vi "Memory.Pointer.External.Encapsulate.vi"(8 "error in (no error)":errorcluster, 10 "size":u64 format="%d bytes", 11 "address":u64 format="%016x") -> (0 "error out":errorcluster, 3 "external pointer":refnum<class "Memory.Pointer.External.lvclass">)   [LabVIEW 2016, in "Memory Manager.lvlib" / "Memory.Pointer.External.lvclass"]
doc: "Encapsulates an existing pointer allocated externally to LabVIEW to allow manipulation of that pointer using this library."
uses:
  Memory.Pointer.External.lvclass
  C:/Users/Ryan/Documents/Git/Sourcetree/LabVIEW-Memory-Manager/Source/Library/Classes/Pointer/Memory.Pointer.lvclass
  Pointer/Memory.Pointer.lvclass/Memory.Pointer.ctl
  Pointer/Methods/Memory.Pointer.Errors.vi
  Pointer/Methods/Memory.Pointer.Errors.Null Pointer.vi
  Pointer/Accessors/Get Address.vi
  Pointer/Methods/Memory.Pointer.Errors.Create Error.vi
  Submodules/Static Error Handling/Source/Library/VIs/Static Error Handling.Error Cluster Constant.vi
  Submodules/Static Error Handling/Source/Library/VIs/Static Error Handling.Error Cluster Constant (256B).vi
  Submodules/Static Error Handling/Source/Library/VIs/Static Error Handling.Parameters.Status.Set.vi
  Submodules/Static Error Handling/Source/Library/VIs/Static Error Handling.Parameters.Code.Set.vi
  Submodules/Static Error Handling/Source/Library/VIs/Static Error Handling.Parameters.VI Source.Set.vi
  Constants/Memory.Constants.vi
  Constants/Memory.Constants.Library Name.vi
  Pointer/Methods/Memory.Pointer.Errors.Get Info.vi
  Submodules/Static Error Handling/Source/Library/VIs/Static Error Handling.Source Buffer.Write.String.vi
  Pointer/Memory.Pointer.lvclass
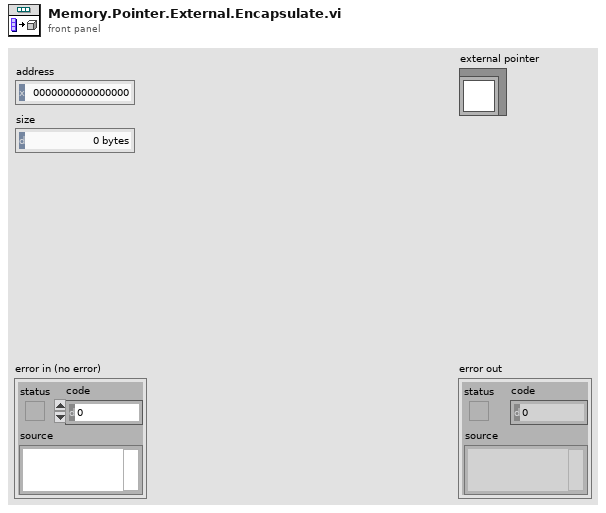
[diagram p1: front panel]
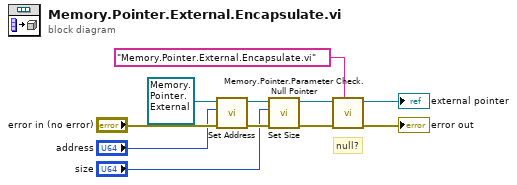
[diagram p0: block diagram]
diagram:
  # "null?"
  n1 = call "Set Address.vi"("error in (no error)"="error in (no error)", "address"="address", "Pointer in"=refnum<class "Memory.Pointer.External.lvclass"> refnum ("pointer out")) -> ("error out"=w8:errorcluster, "Pointer out"=w9:refnum<class "Memory.Pointer.External.lvclass">)  [unwired: 7 in]
  n2 = call "Set Size.vi"("error in (no error)"=w8, "size"="size", "Pointer in"=w9) -> ("error out"=w4:errorcluster, "Pointer out"=w5:refnum<class "Memory.Pointer.External.lvclass">)  [unwired: 7 in]
  n3 = call "Memory.Pointer.Parameter Check.Null Pointer.vi"("source vi name"="Memory.Pointer.External.Encapsulate.vi", "error in (no error)"=w4, "Pointer in"=w5) -> ("error out"=→"error out":errorcluster, "Pointer out"=→"external pointer":refnum<class "Memory.Pointer.External.lvclass">)  [unwired: 7 in]
